vi "Run Filter.vi"(8 "error in (no error)":errorcluster, 10 "resource entries in":T1[](array[typedef]) {"FPGA CD Ref" format="%.0x"; "reserver" format="%.0x"}, 11 "NOT Filter in":refnum<class "NOT Filter.lvclass">) -> (0 "error out":errorcluster, 2 "resource entries out":T1[](array[typedef]) {"FPGA CD Ref" format="%.0x"; "reserver" format="%.0x"})   [LabVIEW 2016, in "FPGA Resource Manager.lvlib" / "NOT Filter.lvclass"]
uses:
  NOT Filter.lvclass
  Server/resource info.ctl
  <vilib>/NI Veristand/Custom Device API/Custom Device Item Ref.ctl
  NOT Filter.lvclass/NOT Filter.ctl
  Filter Parent/Filter.lvclass
  <vilib>/NI VeriStand/Custom Device API/Custom Device API.lvlib
  FPGA Resource Manager.lvlib
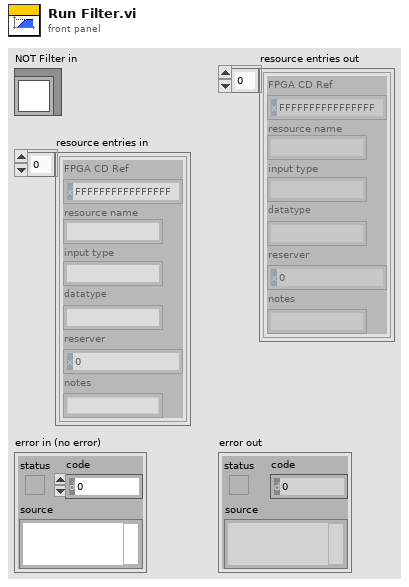
[diagram p1: front panel]
types:
  T1 = typedef "FPGA Resource Manager.lvlib/resource info.ctl" = cluster{"FPGA CD Ref":T2, "resource name":string, "input type":string, "datatype":string, "reserver":T2, "notes":string}
  T2 = typedef "Custom Device API.lvlib/Custom Device Item Ref.ctl" = u64
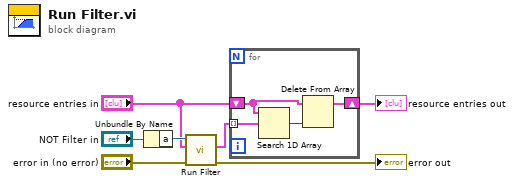
[diagram p0: block diagram]
diagram:
  n1 = Unbundle By Name("NOT Filter in") -> ("a"=w6:refnum<class "Filter.lvclass">)
  n2 = call-dynamic "Run Filter.vi"("error in (no error)"="error in (no error)", "resource entries in"="resource entries in", "Filter in"=w6) -> ("error out"=→"error out":errorcluster, "resource entries out"=w5:T1[])  [unwired: 7 in]
  n3 = for {
    tunnel: w5 -> [w11] mode=indexing
    shift-right: [w8] -> w3
    shift-left: "resource entries in" -> [w10]
    n4 = Search 1D Array(1D array=w10, element=w11) -> (index of element=w9:i32)  [unwired: 1 in]
    n5 = Delete From Array(array=w10, index=w9) -> (array with subset deleted=w8:T1[])  [unwired: 1 in, 1 out]
  }
  "resource entries out" <- w3
